vi "LSMcontroller_v62_updatedpointscan.vi"() -> ()   [LabVIEW 2015] (continued)
                                n1312 = Unbundle By Name(w3824) -> ("autoshutter"=w3823:bool, "wavdet"=w3819:bool)
                                n1313 = case shown="False" w3823 {
                                tunnel: [w3829 w3849] -> w3822
                                tunnel: [w3828 FALSE ("removal")] -> w3821
                                tunnel: [w3827 w3847] -> w3820
                                tunnel: w3819 -> [w3826 _]
                                frame False {
                                n1314 = case shown="False" w3826 {
                                tunnel: [FALSE ("addition") FALSE ("addition")] -> w3829
                                tunnel: [w3831 FALSE ("removal")] -> w3828
                                tunnel: [w3830 _] -> w3827
                                frame False {
                                n1315 = call "configuration.vi"("command"="get") -> ("config out"=w3837:T11)  [unwired: 2 in, 1 out]
                                n1316 = Unbundle By Name(w3837) -> ("2P shutter"=w3834:i32)
                                n1317 = call "2pparameters.vi"("command"="get") -> ("params out"=w3835:T10)  [unwired: 1 in]
                                n1318 = in-place {
                                in-place-border: w3834 -> [w3844]
                                in-place-border: [w3841] -> w3831
                                in-place-border: [w3840] -> w3830
                                n1319 = in-place-cluster #25(w3835) -> ("aDO"=w3843:u32[])
                                n1320 = call "remove channel from active arrayv2.vi"("line array in"=w3843, "line to remove"=w3844) -> ("line array out"=w3842:u32[], "removal"=w3841:bool, "index"=w3840:i32)
                                n1321 = in-place-cluster #25("aDO"=w3842) -> (w3832:T10)
                                }
                                n1322 = call "2pparameters.vi"("Params in"=w3832, "command"="set") -> ()  [unwired: 1 out]
                                }
                                frame True {
                                }
                                }
                                }
                                frame True {
                                n1323 = call "configuration.vi"("command"="get") -> ("config out"=w3851:T11)  [unwired: 2 in, 1 out]
                                n1324 = call "2pparameters.vi"("command"="get") -> ("params out"=w3855:T10)  [unwired: 1 in]
                                n1325 = Unbundle By Name(w3851) -> ("2P shutter"=w3850:i32)
                                n1326 = in-place {
                                in-place-border: w3850 -> [w3861]
                                in-place-border: [w3858] -> w3849
                                in-place-border: [w3857] -> w3847
                                n1327 = in-place-cluster #26(w3855) -> ("aDO"=w3860:u32[])
                                n1328 = call "add channel to active arrayv2.vi"("line array in"=w3860, "line to add"=w3861) -> ("line array out"=w3859:u32[], "addition"=w3858:bool, "index"=w3857:i32)
                                n1329 = in-place-cluster #26("aDO"=w3859) -> (w3853:T10)
                                }
                                n1330 = call "2pparameters.vi"("Params in"=w3853, "command"="set") -> ()  [unwired: 1 out]
                                }
                                }
                                }
                                frame #3 {
                                n1331 = local read "Measurement"() -> (w3865:T4)
                                n1332 = To Unsigned Long Integer(number=w3865) -> (unsigned 32bit integer=w3866:u32)
                                n1333 = case shown="5..7" w3866 {
                                tunnel: [FALSE ("addition") w3884] -> w3864
                                tunnel: [w3869 FALSE ("removal")] -> w3863
                                tunnel: [w3867 w3882] -> w3862
                                frame 0..4, Default {
                                n1334 = call "configuration.vi"("command"="get") -> ("config out"=w3875:T11)  [unwired: 2 in, 1 out]
                                n1335 = Unbundle By Name(w3875) -> ("LT timestamp"=w3872:u32)
                                n1336 = call "2pparameters.vi"("command"="get") -> ("params out"=w3873:T10)  [unwired: 1 in]
                                n1337 = in-place {
                                in-place-border: w3872 -> [w3881]
                                in-place-border: [w3878] -> w3869
                                in-place-border: [w3877] -> w3867
                                n1338 = in-place-cluster #27(w3873) -> ("aDO"=w3880:u32[])
                                n1339 = call "remove channel from active arrayv2.vi"("line array in"=w3880, "line to remove"=w3881) -> ("line array out"=w3879:u32[], "removal"=w3878:bool, "index"=w3877:i32)
                                n1340 = in-place-cluster #27("aDO"=w3879) -> (w3870:T10)
                                }
                                n1341 = call "2pparameters.vi"("Params in"=w3870, "command"="set") -> ()  [unwired: 1 out]
                                }
                                frame 5..7 {
                                n1342 = call "configuration.vi"("command"="get") -> ("config out"=w3890:T11)  [unwired: 2 in, 1 out]
                                n1343 = Unbundle By Name(w3890) -> ("LT timestamp"=w3887:u32)
                                n1344 = call "2pparameters.vi"("command"="get") -> ("params out"=w3888:T10)  [unwired: 1 in]
                                n1345 = in-place {
                                in-place-border: w3887 -> [w3896]
                                in-place-border: [w3893] -> w3884
                                in-place-border: [w3892] -> w3882
                                n1346 = in-place-cluster #28(w3888) -> ("aDO"=w3895:u32[])
                                n1347 = call "add channel to active arrayv2.vi"("line array in"=w3895, "line to add"=w3896) -> ("line array out"=w3894:u32[], "addition"=w3893:bool, "index"=w3892:i32)
                                n1348 = in-place-cluster #28("aDO"=w3894) -> (w3885:T10)
                                }
                                n1349 = call "2pparameters.vi"("Params in"=w3885, "command"="set") -> ()  [unwired: 1 out]
                                }
                                }
                                }
                                }
                                }
                                frame #1 {
                                n1350 = Or(x=w3903, y=w3904) -> (x .or. y?=w3902:bool)
                                n1351 = case shown="True" w3902 {
                                frame False {
                                }
                                frame True {
                                # "update GUI"
                                n1352 = call "Used AO lines.vi"() -> ("used AO names"=w3908:string[], "used AO lines"=w3910:tag[])  [unwired: 2 in]
                                n1353 = control-ref of="Analog Lines Plot"() -> (w3909:refnum<vi>)
                                n1354 = local write "Analog Used Lines"(w3910) -> ()
                                n1355 = local write "Analog Used Names"(w3908) -> ()
                                n1356 = call "prepAOWaveplot.vi"("WaveformGraph in"=w3909, "Analog Used Names"=w3908) -> ()  [unwired: 1 in]
                                }
                                }
                                n1357 = Compound Arithmetic op=OR(w3900, w3899, w3898, w3897) -> (w3901:bool)
                                n1358 = case shown="True" w3901 {
                                frame False {
                                }
                                frame True {
                                n1359 = control-ref of="Digital Lines Plot"() -> (w3905:refnum<vi>)
                                n1360 = call "Used DO lines.vi"() -> ("used DO names"=w3906:string[], "used DO lines"=w3907:tag[])  [unwired: 2 in]
                                n1361 = local write "Digital Used Lines"(w3907) -> ()
                                n1362 = local write "Digital Used Names"(w3906) -> ()
                                n1363 = call "prepDOWaveplot.vi"("DigitalGraph in"=w3905, "used DO names"=w3906) -> ()  [unwired: 1 in]
                                }
                                }
                                }
                                frame #2 {
                                n1364 = case shown="False" w3914 {
                                tunnel: [w3917 w3943] -> w3913
                                tunnel: [w3916 w3941] -> w3912
                                tunnel: [w3915 _] -> w3911
                                frame False {
                                n1365 = stacked-sequence {
                                seq-local: [w3919 _] -> [_ w3934]
                                tunnel: [w3919 _] -> w3917
                                tunnel: [w3922 _] -> w3916
                                tunnel: [w3918 _] -> w3915
                                frame #0 {
                                n1366 = call "configuration.vi"("command"="get") -> ("config out"=w3930:T11)  [unwired: 2 in, 1 out]
                                n1367 = call "waveformparamsv2.vi"("command"="get") -> ("Params out"=w3924:T14)  [unwired: 4 in, 2 out]
                                n1368 = Unbundle By Name(w3930) -> ("Voltage to Xgalvo"=w3931:i32)
                                n1369 = call "2pparameters.vi"("command"="get") -> ("params out"=w3927:T10)  [unwired: 1 in]
                                n1370 = Unbundle By Name(w3924) -> ("AO parameters"=w3923:T15)
                                n1371 = Unbundle By Name(w3927) -> ("aAO"=w3928:u32[])
                                n1372 = call "waveformsAObuffer.vi"("command"="get") -> ("AO wf out"=w3920:waveform(dbl)[])  [unwired: 1 in]
                                n1373 = Search 1D Array(1D array=w3928, element=w3931) -> (index of element=w3919:i32)  [unwired: 1 in]
                                n1374 = Index Array(array=w3920, index=w3919) -> (element=w3918:waveform(dbl))
                                n1375 = Index Array(array=w3923, index=w3919) -> (element=w3922:T16)
                                }
                                frame #1 {
                                w3935 = 0.0 ("Step size (V)")
                                n1376 = local read "Meastab"() -> (w3933:enum32{"X-Y Image", "Linescan", "Timetrace"})
                                n1377 = case shown="\"X-Y Image\", Default" w3933 {
                                tunnel: [w3937 w3938] -> w3932
                                frame "X-Y Image", Default {
                                n1378 = local read "Sampling rate"() -> (w3937:dbl)
                                }
                                frame "Timetrace" {
                                n1379 = local read "srateAODOtt"() -> (w3938:dbl)
                                }
                                }
                                n1380 = call "replace AO XYwfparam.vi"("Baseline (V)"=w3935, "Start amplitude (V)"=w3935, "Cycles"=w3935, "Repeats"=w3935, "index of AO wave"=w3934, "Step size (V)"=w3935, "DC (%)"=w3935, "Sampling frequency (Hz)"=w3932, "Period (ms)"=w3935, "Cycle length (s)"=w3935, "Pulses"=w3935, "padding value"=w3935, "Matlab wave name"=path "xwave") -> ()  [unwired: 3 in]
                                }
                                }
                                }
                                frame True {
                                w3942 = 0.0 ("Repeats")
                                n1381 = local read "Meastab"() -> (w3940:enum32{"X-Y Image", "Linescan", "Timetrace"})
                                n1382 = case shown="\"X-Y Image\", Default" w3940 {
                                tunnel: [w3959 w3960] -> w3939
                                frame "X-Y Image", Default {
                                n1383 = local read "Sampling rate"() -> (w3959:dbl)
                                }
                                frame "Timetrace" {
                                n1384 = local read "srateAODOtt"() -> (w3960:dbl)
                                }
                                }
                                n1385 = call "2pparameters.vi"("command"="get") -> ("params out"=w3945:T10)  [unwired: 1 in]
                                n1386 = call "configuration.vi"("command"="get") -> ("config out"=w3948:T11)  [unwired: 2 in, 1 out]
                                n1387 = call "waveformparamsv2.vi"("command"="get") -> ("Params out"=w3956:T14)  [unwired: 4 in, 2 out]
                                n1388 = Unbundle By Name(w3948) -> ("Voltage to Xgalvo"=w3949:i32)
                                n1389 = Unbundle By Name(w3956) -> ("AO parameters"=w3953:T15)
                                n1390 = Unbundle By Name(w3945) -> ("aAO"=w3946:u32[])
                                n1391 = Search 1D Array(1D array=w3946, element=w3949) -> (index of element=w3943:i32)  [unwired: 1 in]
                                n1392 = Index Array(array=w3953, index=0) -> (element=w3954:T16)
                                n1393 = Bundle By Name(cluster=w3954, "AOtab"=-1.0 ("Repeats"), "Repeats"=w3942, "Cycles"=w3942, "Start amplitude (V)"=w3942, "Baseline (V)"=w3942, "Step size (V)"=w3942, "DC (%)"=w3942, "Sampling frequency (Hz)"=w3939, "Period (ms)"=w3942, "Offset (V)"=w3942, "Amplitude (V)"=w3942, "Frequency"=w3942, "Tri Repeats"=w3942, "phase shift (ms)"=w3942, "Pulses"=w3942, "Matlab wave file"=path "xwave", "padding value"=w3942) -> (w3941:T16)
                                n1394 = Build Array(w3941) -> (w3951:T15)
                                n1395 = call "waveformparamsv2.vi"("command"="add AO", "add AO"=w3951) -> ()  [unwired: 3 in, 3 out]
                                }
                                }
                                }
                                frame #3 {
                                n1396 = case shown="False" w3964 {
                                tunnel: [w3967 w3993] -> w3963
                                tunnel: [w3966 w3991] -> w3962
                                tunnel: [w3965 _] -> w3961
                                frame False {
                                n1397 = stacked-sequence {
                                seq-local: [w3969 _] -> [_ w3984]
                                tunnel: [w3969 _] -> w3967
                                tunnel: [w3972 _] -> w3966
                                tunnel: [w3968 _] -> w3965
                                frame #0 {
                                n1398 = call "configuration.vi"("command"="get") -> ("config out"=w3980:T11)  [unwired: 2 in, 1 out]
                                n1399 = call "waveformparamsv2.vi"("command"="get") -> ("Params out"=w3974:T14)  [unwired: 4 in, 2 out]
                                n1400 = Unbundle By Name(w3980) -> ("Voltage to Ygalvo"=w3981:i32)
                                n1401 = call "2pparameters.vi"("command"="get") -> ("params out"=w3977:T10)  [unwired: 1 in]
                                n1402 = Unbundle By Name(w3974) -> ("AO parameters"=w3973:T15)
                                n1403 = Unbundle By Name(w3977) -> ("aAO"=w3978:u32[])
                                n1404 = call "waveformsAObuffer.vi"("command"="get") -> ("AO wf out"=w3970:waveform(dbl)[])  [unwired: 1 in]
                                n1405 = Search 1D Array(1D array=w3978, element=w3981) -> (index of element=w3969:i32)  [unwired: 1 in]
                                n1406 = Index Array(array=w3970, index=w3969) -> (element=w3968:waveform(dbl))
                                n1407 = Index Array(array=w3973, index=w3969) -> (element=w3972:T16)
                                }
                                frame #1 {
                                w3985 = 0.0 ("Step size (V)")
                                n1408 = local read "Meastab"() -> (w3983:enum32{"X-Y Image", "Linescan", "Timetrace"})
                                n1409 = case shown="\"X-Y Image\", Default" w3983 {
                                tunnel: [w3987 w3988] -> w3982
                                frame "X-Y Image", Default {
                                n1410 = local read "Sampling rate"() -> (w3987:dbl)
                                }
                                frame "Timetrace" {
                                n1411 = local read "srateAODOtt"() -> (w3988:dbl)
                                }
                                }
                                n1412 = call "replace AO XYwfparam.vi"("Baseline (V)"=w3985, "Start amplitude (V)"=w3985, "Cycles"=w3985, "Repeats"=w3985, "index of AO wave"=w3984, "Step size (V)"=w3985, "DC (%)"=w3985, "Sampling frequency (Hz)"=w3982, "Period (ms)"=w3985, "Cycle length (s)"=w3985, "Pulses"=w3985, "padding value"=w3985, "Matlab wave name"=path "ywave") -> ()  [unwired: 3 in]
                                }
                                }
                                }
                                frame True {
                                w3992 = 0.0 ("Repeats")
                                n1413 = local read "Meastab"() -> (w3990:enum32{"X-Y Image", "Linescan", "Timetrace"})
                                n1414 = case shown="\"X-Y Image\", Default" w3990 {
                                tunnel: [w4009 w4010] -> w3989
                                frame "X-Y Image", Default {
                                n1415 = local read "Sampling rate"() -> (w4009:dbl)
                                }
                                frame "Timetrace" {
                                n1416 = local read "srateAODOtt"() -> (w4010:dbl)
                                }
                                }
                                n1417 = call "2pparameters.vi"("command"="get") -> ("params out"=w3995:T10)  [unwired: 1 in]
                                n1418 = call "configuration.vi"("command"="get") -> ("config out"=w3998:T11)  [unwired: 2 in, 1 out]
                                n1419 = call "waveformparamsv2.vi"("command"="get") -> ("Params out"=w4007:T14)  [unwired: 4 in, 2 out]
                                n1420 = Unbundle By Name(w3998) -> ("Voltage to Ygalvo"=w3999:i32)
                                n1421 = Unbundle By Name(w4007) -> ("AO parameters"=w4004:T15)
                                n1422 = Unbundle By Name(w3995) -> ("aAO"=w3996:u32[])
                                n1423 = Search 1D Array(1D array=w3996, element=w3999) -> (index of element=w3993:i32)  [unwired: 1 in]
                                n1424 = Index Array(array=w4004, index=0) -> (element=w4005:T16)
                                n1425 = Bundle By Name(cluster=w4005, "AOtab"=-1.0 ("Repeats"), "Repeats"=w3992, "Cycles"=w3992, "Start amplitude (V)"=w3992, "Baseline (V)"=w3992, "Step size (V)"=w3992, "DC (%)"=w3992, "Sampling frequency (Hz)"=w3989, "Period (ms)"=w3992, "Offset (V)"=w3992, "Amplitude (V)"=w3992, "Frequency"=w3992, "Tri Repeats"=w3992, "phase shift (ms)"=w3992, "Pulses"=w3992, "Matlab wave file"=path "ywave", "padding value"=w3992) -> (w3991:T16)
                                n1426 = Build Array(w3991) -> (w4002:T15)
                                n1427 = call "waveformparamsv2.vi"("command"="add AO", "add AO"=w4002) -> ()  [unwired: 3 in, 3 out]
                                }
                                }
                                }
                                frame #4 {
                                n1428 = call "2pparameters.vi"("command"="get") -> ("params out"=w4016:T10)  [unwired: 1 in]
                                n1429 = Unbundle By Name(w4016) -> ("wavdet"=w4015:bool, "Pel"=w4012:sgl, "refwfsize"=w4011:dbl, "srateAODO"=w4014:sgl)
                                n1430 = case shown="True" w4015 {
                                tunnel: [w4020 w4030] -> w4018
                                tunnel: w4014 -> [w4021 w4032]
                                tunnel: w4012 -> [_ w4028]
                                tunnel: w4011 -> [_ w4027]
                                frame False {
                                n1431 = call "X-array-databuffer.vi"("command"=enum16{"get", "set", "clear", "append"}."get") -> ("array out"=w4024:dbl[])  [unwired: 3 in, 1 out]
                                n1432 = Reciprocal(x=w4021) -> (1/x=w4022:sgl)
                                n1433 = Bundle By Name("Y"=w4024, "dt"=w4022) -> (w4020:waveform(dbl))  [unwired: 1 in]
                                }
                                frame True {
                                n1434 = To Double Precision Float(number=w4028) -> (double precision float=w4029:dbl)
                                n1435 = Divide(x=w4027, y=w4029) -> (x/y=w4026:dbl)
                                n1436 = Round Toward +Infinity(x=w4026) -> (ceil(x): smallest int >= x=w4025:dbl)
                                n1437 = call "X-array-databuffer.vi"("command"=enum16{"get", "set", "clear", "append"}."get") -> ("array out"=w4034:dbl[])  [unwired: 3 in, 1 out]
                                n1438 = Reciprocal(x=w4032) -> (1/x=w4033:sgl)
                                n1439 = for {
                                N: w4025 -> [_]
                                tunnel: w4034 -> [w4036]
                                tunnel: [w4036] -> w4031 mode=concatenating
                                }
                                n1440 = Bundle By Name("Y"=w4031, "dt"=w4033) -> (w4030:waveform(dbl))  [unwired: 1 in]
                                }
                                }
                                n1441 = case shown="True" w4019 {
                                tunnel: w4018 -> [w4038 w4044]
                                tunnel: w4013 -> [w4039 _]
                                frame False {
                                n1442 = call "waveformsAObuffer.vi"("command"="get") -> ("AO wf out"=w4042:waveform(dbl)[])  [unwired: 1 in]
                                n1443 = property on="refwf" class="Ring (strict)" props=["RingText", "Text"]() -> ()  [unwired: 2 in, 3 out]
                                n1444 = Replace Array Subset(array=w4042, new element=w4038, index=w4039) -> (w4037:waveform(dbl)[])
                                n1445 = call "waveformsAObuffer.vi"("AO wf in"=w4037, "command"="set") -> ()  [unwired: 1 out]
                                }
                                frame True {
                                n1446 = call "waveformsAObuffer.vi"("command"="get") -> ("AO wf out"=w4046:waveform(dbl)[])  [unwired: 1 in]
                                n1447 = Build Array (concatenate)(w4046, w4044) -> (w4043:waveform(dbl)[])
                                n1448 = call "waveformsAObuffer.vi"("AO wf in"=w4043, "command"="set") -> ()  [unwired: 1 out]
                                }
                                }
                                }
                                frame #5 {
                                n1449 = call "2pparameters.vi"("command"="get") -> ("params out"=w4058:T10)  [unwired: 1 in]
                                n1450 = Unbundle By Name(w4058) -> ("wavdet"=w4057:bool, "Pel"=w4055:sgl, "refwfsize"=w4056:dbl, "srateAODO"=w4051:sgl)
                                n1451 = To Double Precision Float(number=w4055) -> (double precision float=w4054:dbl)
                                n1452 = Divide(x=w4056, y=w4054) -> (x/y=w4053:dbl)
                                n1453 = Round Toward +Infinity(x=w4053) -> (ceil(x): smallest int >= x=w4052:dbl)
                                n1454 = case shown="True" w4057 {
                                tunnel: [w4062 w4068] -> w4048
                                tunnel: w4052 -> [_ w4065]
                                tunnel: w4051 -> [w4063 w4070]
                                frame False {
                                n1455 = call "Y-array-databuffer.vi"("command"=enum16{"get", "set", "clear", "append"}."get") -> ("array out"=w4060:dbl[])  [unwired: 3 in, 1 out]
                                n1456 = Reciprocal(x=w4063) -> (1/x=w4064:sgl)
                                n1457 = Bundle By Name("Y"=w4060, "dt"=w4064) -> (w4062:waveform(dbl))  [unwired: 1 in]
                                }
                                frame True {
                                n1458 = call "Y-array-databuffer.vi"("command"=enum16{"get", "set", "clear", "append"}."get") -> ("array out"=w4066:dbl[])  [unwired: 3 in, 1 out]
                                n1459 = Reciprocal(x=w4070) -> (1/x=w4071:sgl)
                                n1460 = for {
                                N: w4065 -> [_]
                                tunnel: w4066 -> [w4072]
                                tunnel: [w4072] -> w4069 mode=concatenating
                                }
                                n1461 = Bundle By Name("Y"=w4069, "dt"=w4071) -> (w4068:waveform(dbl))  [unwired: 1 in]
                                }
                                }
                                n1462 = case shown="False" w4050 {
                                tunnel: w4048 -> [w4075 w4080]
                                tunnel: w4049 -> [w4076 _]
                                frame False {
                                n1463 = call "waveformsAObuffer.vi"("command"="get") -> ("AO wf out"=w4078:waveform(dbl)[])  [unwired: 1 in]
                                n1464 = Replace Array Subset(array=w4078, new element=w4075, index=w4076) -> (w4073:waveform(dbl)[])
                                n1465 = call "waveformsAObuffer.vi"("AO wf in"=w4073, "command"="set") -> ()  [unwired: 1 out]
                                }
                                frame True {
                                n1466 = call "waveformsAObuffer.vi"("command"="get") -> ("AO wf out"=w4082:waveform(dbl)[])  [unwired: 1 in]
                                n1467 = Build Array (concatenate)(w4082, w4080) -> (w4079:waveform(dbl)[])
                                n1468 = call "waveformsAObuffer.vi"("AO wf in"=w4079, "command"="set") -> ()  [unwired: 1 out]
                                }
                                }
                                }
                                frame #6 {
                                n1469 = Build Array(w4087, w4086) -> (w4090:bool[])
                                n1470 = Boolean Array To Number(Boolean array=w4090) -> (number=w4089:u32)
                                n1471 = case shown="2" w4089 {
                                tunnel: w4088 -> [_ _ _ _]
                                tunnel: w4085 -> [_ w4113 _ w4126]
                                tunnel: [_ w4112 _ w4123] -> w4084
                                frame 1 {
                                w4100 = 0.0 ("DOtab")
                                n1472 = call "2pparameters.vi"("command"="get") -> ("params out"=w4097:T10)  [unwired: 1 in]
                                n1473 = call "waveformparamsv2.vi"("command"="get") -> ("Params out"=w4108:T14)  [unwired: 4 in, 2 out]
                                n1474 = Unbundle By Name(w4108) -> ("DO parameters"=w4106:T17)
                                n1475 = Unbundle By Name(w4097) -> ("srate"=w4093:sgl, "Pel"=w4096:sgl)
                                n1476 = To Double Precision Float(number=w4093) -> (double precision float=w4091:dbl)
                                n1477 = To Double Precision Float(number=w4093) -> (double precision float=w4092:dbl)
                                n1478 = To Double Precision Float(number=w4096) -> (double precision float=w4095:dbl)
                                n1479 = Divide(x=w4092, y=w4095) -> (x/y=w4094:dbl)
                                n1480 = Index Array(array=w4106, index=0) -> (element=w4105:T18)
                                n1481 = Bundle By Name(cluster=w4105, "Digital DC (%)"=100.0, "Digital phase"=w4100, "Digital Freq (Hz)"=w4094, "Sampling frequency (Hz)"=w4091, "Digital time offset (s)"=w4100, "padding value"=0.0, "matlab wave file"=path "2Pshutter", "DOtab"=0.0) -> (w4103:T18)
                                n1482 = Build Array(w4103) -> (w4102:T17)
                                n1483 = call "waveformparamsv2.vi"("command"="add DO", "add DO"=w4102) -> ()  [unwired: 3 in, 3 out]
                                }
                                frame 2 {
                                n1484 = call "waveformparamsv2.vi"("command"="get") -> ("Params out"=w4115:T14)  [unwired: 4 in, 2 out]
                                n1485 = in-place {
                                in-place-border: w4113 -> [w4119]
                                in-place-border: [w4118] -> w4112
                                n1486 = in-place-cluster #29(w4115) -> ("DO parameters"=w4121:T17)
                                n1487 = Delete From Array(array=w4121, length=1, index=w4119) -> (deleted portion=w4118:T17, array with subset deleted=w4120:T17)
                                n1488 = in-place-cluster #29("DO parameters"=w4120) -> (w4114:T14)
                                }
                                n1489 = call "waveformparamsv2.vi"("command"="set", "Params in"=w4114) -> ()  [unwired: 3 in, 3 out]
                                }
                                frame 3, Default {
                                }
                                frame 0 {
                                n1490 = call "2pparameters.vi"("command"="get") -> ("params out"=w4128:T10)  [unwired: 1 in]
                                n1491 = Unbundle By Name(w4128) -> ("wavdet"=w4125:bool, "autoshutter"=w4127:bool)
                                n1492 = case shown="True" w4127 {
                                tunnel: w4126 -> [_ w4132]
                                tunnel: w4125 -> [_ w4131]
                                tunnel: [_ w4130] -> w4124
                                frame False {
                                }
                                frame True {
                                n1493 = case shown="False" w4131 {
                                tunnel: w4132 -> [w4134 _]
                                tunnel: [w4133 _] -> w4130
                                frame False {
                                n1494 = stacked-sequence {
                                tunnel: w4134 -> [w4136 w4150]
                                tunnel: [w4135 _] -> w4133
                                frame #0 {
                                n1495 = call "waveformparamsv2.vi"("command"="get") -> ("Params out"=w4138:T14)  [unwired: 4 in, 2 out]
                                n1496 = Unbundle By Name(w4138) -> ("DO parameters"=w4137:T17)
                                n1497 = Index Array(array=w4137, index=w4136) -> (element=w4135:T18)
                                }
                                frame #1 {
                                w4149 = 0.0 ("padding value")
                                n1498 = call "2pparameters.vi"("command"="get") -> ("params out"=w4147:T10)  [unwired: 1 in]
                                n1499 = Unbundle By Name(w4147) -> ("srate"=w4144:sgl, "Pel"=w4146:sgl)
                                n1500 = To Double Precision Float(number=w4144) -> (double precision float=w4142:dbl)
                                n1501 = To Double Precision Float(number=w4144) -> (double precision float=w4143:dbl)
                                n1502 = To Double Precision Float(number=w4146) -> (double precision float=w4145:dbl)
                                n1503 = Divide(x=w4143, y=w4145) -> (x/y=w4141:dbl)
                                n1504 = call "replace DO wf param.vi"("Digital Freq (Hz)"=w4141, "Digital DC (%)"=100.0, "Digital phase"=w4149, "Sampling frequency (Hz)"=w4142, "Digital time offset (s)"=w4149, "index of DO wave"=w4150, "padding value"=w4149, "matlab wave file"=path "2Pshutter" ("matlab wave number")) -> ()  [unwired: 3 in]
                                }
                                }
                                }
                                frame True {
                                }
                                }
                                }
                                }
                                n1505 = Build Array(w4124) -> (w4123:T17)
                                }
                                }
                                }
                                frame #7 {
                                n1506 = Build Array(w4155, w4154) -> (w4157:bool[])
                                n1507 = Boolean Array To Number(Boolean array=w4157) -> (number=w4156:u32)
                                n1508 = case shown="0" w4156 {
                                tunnel: w4153 -> [_ w4199 _ w4206]
                                tunnel: [_ w4198 _ w4204] -> w4152
                                frame 1 {
                                n1509 = call "2pparameters.vi"("command"="get") -> ("params out"=w4164:T10)  [unwired: 1 in]
                                n1510 = Unbundle By Name(w4164) -> ("wavdet"=w4165:bool, "Pel"=w4167:sgl, "refwfsize"=w4168:dbl, "srateAODO"=w4166:sgl)
                                n1511 = call "waveformsDObuffer.vi"("command"="get") -> ("DO wf out"=w4160:digitalwaveform[])  [unwired: 1 in]
                                n1512 = case shown="False" w4165 {
                                tunnel: [w4173 w4183] -> w4162
                                tunnel: w4166 -> [w4178 w4194]
                                tunnel: w4167 -> [w4172 w4187]
                                tunnel: w4168 -> [_ w4191]
                                frame False {
                                w4176 = u16 0 items=["unsigned binary", "offset binary", "2's complement"] ("data format (offset binary)")
                                n1513 = Initialize Array(sgl 1.0, w4172) -> (w4169:sgl[])
                                n1514 = Reciprocal(x=w4178) -> (1/x=w4179:sgl)
                                n1515 = Bundle By Name("Y"=w4169, "dt"=w4179) -> (w4174:waveform(sgl))  [unwired: 1 in]
                                n1516 = call-poly <vilib>:"Analog to Digital.vi"("data format (offset binary)"=w4176, "compress digital (T)"=TRUE, "full-scale range (pk-pk)"=1.0, "resolution (16 bit)"=1, "analog waveform"=w4174) -> ("digital waveform"=w4173:digitalwaveform)  [unwired: 3 in, 3 out]
                                }
                                frame True {
                                w4186 = u16 0 items=["unsigned binary", "offset binary", "2's complement"] ("data format (offset binary)")
                                n1517 = To Double Precision Float(number=w4187) -> (double precision float=w4192:dbl)
                                n1518 = Initialize Array(sgl 1.0, w4187) -> (w4180:sgl[])
                                n1519 = Divide(x=w4191, y=w4192) -> (x/y=w4189:dbl)
                                n1520 = Round Toward +Infinity(x=w4189) -> (ceil(x): smallest int >= x=w4190:dbl)
                                n1521 = for {
                                N: w4190 -> [_]
                                tunnel: w4180 -> [w4196]
                                tunnel: [w4196] -> w4193 mode=concatenating
                                }
                                n1522 = Reciprocal(x=w4194) -> (1/x=w4195:sgl)
                                n1523 = Bundle By Name("Y"=w4193, "dt"=w4195) -> (w4184:waveform(sgl))  [unwired: 1 in]
                                n1524 = call-poly <vilib>:"Analog to Digital.vi"("data format (offset binary)"=w4186, "compress digital (T)"=TRUE, "full-scale range (pk-pk)"=1.0, "resolution (16 bit)"=1, "analog waveform"=w4184) -> ("digital waveform"=w4183:digitalwaveform)  [unwired: 3 in, 3 out]
                                }
                                }
                                n1525 = Build Array (concatenate)(w4160, w4162) -> (w4158:digitalwaveform[])
                                n1526 = call "waveformsDObuffer.vi"("DO wf in"=w4158, "command"="set") -> ()  [unwired: 1 out]
                                }
                                frame 2 {
                                n1527 = call "waveformsDObuffer.vi"("command"="get") -> ("DO wf out"=w4201:digitalwaveform[])  [unwired: 1 in]
                                n1528 = Delete From Array(array=w4201, length=1, index=w4199) -> (deleted portion=w4198:digitalwaveform[], array with subset deleted=w4197:digitalwaveform[])
                                n1529 = call "waveformsDObuffer.vi"("DO wf in"=w4197, "command"="set") -> ()  [unwired: 1 out]
                                }
                                frame 3, Default {
                                }
                                frame 0 {
                                n1530 = call "2pparameters.vi"("command"="get") -> ("params out"=w4208:T10)  [unwired: 1 in]
                                n1531 = Unbundle By Name(w4208) -> ("autoshutter"=w4207:bool, "wavdet"=w4205:bool)
                                n1532 = case shown="True" w4207 {
                                tunnel: w4206 -> [_ w4212]
                                tunnel: w4205 -> [_ w4211]
                                tunnel: [_ w4210] -> w4204
                                frame False {
                                }
                                frame True {
                                n1533 = case shown="False" w4211 {
                                tunnel: w4212 -> [w4216 _]
                                tunnel: [w4214 _] -> w4210
                                frame False {
                                w4223 = u16 0 items=["unsigned binary", "offset binary", "2's complement"] ("data format (offset binary)")
                                n1534 = call "2pparameters.vi"("command"="get") -> ("params out"=w4230:T10)  [unwired: 1 in]
                                n1535 = call "waveformsDObuffer.vi"("command"="get") -> ("DO wf out"=w4217:digitalwaveform[])  [unwired: 1 in]
                                n1536 = Unbundle By Name(w4230) -> ("Pel"=w4232:sgl, "srate"=w4231:sgl)
                                n1537 = Index Array(array=w4217, index=w4216) -> (element=w4215:digitalwaveform)
                                n1538 = Build Array(w4215) -> (w4214:digitalwaveform[])
                                n1539 = Initialize Array(sgl 1.0, w4232) -> (w4218:sgl[])
                                n1540 = Reciprocal(x=w4231) -> (1/x=w4225:sgl)
                                n1541 = Bundle By Name("Y"=w4218, "dt"=w4225) -> (w4221:waveform(sgl))  [unwired: 1 in]
                                n1542 = call-poly <vilib>:"Analog to Digital.vi"("data format (offset binary)"=w4223, "compress digital (T)"=TRUE, "full-scale range (pk-pk)"=1.0, "resolution (16 bit)"=1, "analog waveform"=w4221) -> ("digital waveform"=w4228:digitalwaveform)  [unwired: 3 in, 3 out]
                                n1543 = Replace Array Subset(array=w4217, new element=w4228, index=w4216) -> (w4213:digitalwaveform[])
                                n1544 = call "waveformsDObuffer.vi"("DO wf in"=w4213, "command"="set") -> ()  [unwired: 1 out]
                                }
                                frame True {
                                }
                                }
                                }
                                }
                                }
                                }
                                }
                                frame #8 {
                                n1545 = Build Array(w4236, w4235) -> (w4238:bool[])
                                n1546 = Boolean Array To Number(Boolean array=w4238) -> (number=w4237:u32)
                                n1547 = case shown="0" w4237 {
                                tunnel: w4234 -> [_ w4264 _ w4276]
                                tunnel: [_ w4263 _ w4274] -> w4233
                                frame 1 {
                                w4251 = 0.0 ("DOtab")
                                n1548 = call "2pparameters.vi"("command"="get") -> ("params out"=w4249:T10)  [unwired: 1 in]
                                n1549 = call "waveformparamsv2.vi"("command"="get") -> ("Params out"=w4259:T14)  [unwired: 4 in, 2 out]
                                n1550 = Unbundle By Name(w4259) -> ("DO parameters"=w4257:T17)
                                n1551 = Unbundle By Name(w4249) -> ("srate"=w4246:sgl, "Pel"=w4248:sgl)
                                n1552 = To Double Precision Float(number=w4246) -> (double precision float=w4244:dbl)
                                n1553 = To Double Precision Float(number=w4246) -> (double precision float=w4245:dbl)
                                n1554 = To Double Precision Float(number=w4248) -> (double precision float=w4240:dbl)
                                n1555 = Divide(x=w4245, y=w4240) -> (x/y=w4247:dbl)
                                n1556 = Index Array(array=w4257, index=0) -> (element=w4256:T18)
                                n1557 = Divide(x=1.0 ("Digital DC (%)"), y=w4240) -> (x/y=w4242:dbl)
                                n1558 = Multiply(x=100.0, y=w4242) -> (x*y=w4239:dbl)
                                n1559 = Bundle By Name(cluster=w4256, "Digital DC (%)"=w4239, "Digital phase"=w4251, "Digital Freq (Hz)"=w4247, "Sampling frequency (Hz)"=w4244, "Digital time offset (s)"=w4251, "padding value"=0.0, "matlab wave file"=path "LT", "DOtab"=0.0) -> (w4254:T18)
                                n1560 = Build Array(w4254) -> (w4253:T17)
                                n1561 = call "waveformparamsv2.vi"("command"="add DO", "add DO"=w4253) -> ()  [unwired: 3 in, 3 out]
                                }
                                frame 2 {
                                n1562 = call "waveformparamsv2.vi"("command"="get") -> ("Params out"=w4266:T14)  [unwired: 4 in, 2 out]
                                n1563 = in-place {
                                in-place-border: w4264 -> [w4270]
                                in-place-border: [w4269] -> w4263
                                n1564 = in-place-cluster #30(w4266) -> ("DO parameters"=w4272:T17)
                                n1565 = Delete From Array(array=w4272, length=1, index=w4270) -> (deleted portion=w4269:T17, array with subset deleted=w4271:T17)
                                n1566 = in-place-cluster #30("DO parameters"=w4271) -> (w4265:T14)
                                }
                                n1567 = call "waveformparamsv2.vi"("command"="set", "Params in"=w4265) -> ()  [unwired: 3 in, 3 out]
                                }
                                frame 3, Default {
                                }
                                frame 0 {
                                n1568 = local read "Measurement"() -> (w4278:T4)
                                n1569 = To Unsigned Long Integer(number=w4278) -> (unsigned 32bit integer=w4277:u32)
                                n1570 = case shown="5..7" w4277 {
                                tunnel: w4276 -> [_ w4280]
                                tunnel: [_ w4279] -> w4275
                                frame 0..4, Default {
                                }
                                frame 5..7 {
                                n1571 = stacked-sequence {
                                tunnel: w4280 -> [w4282 w4291]
                                tunnel: [w4281 _] -> w4279
                                frame #0 {
                                n1572 = call "waveformparamsv2.vi"("command"="get") -> ("Params out"=w4284:T14)  [unwired: 4 in, 2 out]
                                n1573 = Unbundle By Name(w4284) -> ("DO parameters"=w4285:T17)
                                n1574 = Index Array(array=w4285, index=w4282) -> (element=w4281:T18)
                                }
                                frame #1 {
                                w4299 = 0.0 ("padding value")
                                n1575 = call "2pparameters.vi"("command"="get") -> ("params out"=w4297:T10)  [unwired: 1 in]
                                n1576 = Unbundle By Name(w4297) -> ("srate"=w4295:sgl, "Pel"=w4296:sgl)
                                n1577 = To Double Precision Float(number=w4295) -> (double precision float=w4293:dbl)
                                n1578 = To Double Precision Float(number=w4295) -> (double precision float=w4294:dbl)
                                n1579 = To Double Precision Float(number=w4296) -> (double precision float=w4289:dbl)
                                n1580 = Divide(x=1.0 ("Digital DC (%)"), y=w4289) -> (x/y=w4288:dbl)
                                n1581 = Multiply(x=100.0, y=w4288) -> (x*y=w4287:dbl)
                                n1582 = Divide(x=w4294, y=w4289) -> (x/y=w4292:dbl)
                                n1583 = call "replace DO wf param.vi"("Digital Freq (Hz)"=w4292, "Digital DC (%)"=w4287, "Digital phase"=w4299, "Sampling frequency (Hz)"=w4293, "Digital time offset (s)"=w4299, "index of DO wave"=w4291, "padding value"=w4299, "matlab wave file"=path "LT" ("matlab wave number")) -> ()  [unwired: 3 in]
                                }
                                }
                                }
                                }
                                n1584 = Build Array(w4275) -> (w4274:T17)
                                }
                                }
                                }
                                frame #9 {
                                n1585 = Build Array(w4304, w4303) -> (w4306:bool[])
                                n1586 = Boolean Array To Number(Boolean array=w4306) -> (number=w4305:u32)
                                n1587 = case shown="0" w4305 {
                                tunnel: w4302 -> [_ w4358 _ w4362]
                                tunnel: [_ w4353 _ w4359] -> w4301
                                frame 1 {
                                n1588 = call "2pparameters.vi"("command"="get") -> ("params out"=w4313:T10)  [unwired: 1 in]
                                n1589 = Unbundle By Name(w4313) -> ("wavdet"=w4314:bool, "Pel"=w4316:sgl, "refwfsize"=w4317:dbl, "Pel"=w4315:sgl)
                                n1590 = call "waveformsDObuffer.vi"("command"="get") -> ("DO wf out"=w4309:digitalwaveform[])  [unwired: 1 in]
                                n1591 = case shown="True" w4314 {
                                tunnel: [w4321 w4334] -> w4311
                                tunnel: w4315 -> [w4330 w4349]
                                tunnel: w4316 -> [w4320 w4340]
                                tunnel: w4317 -> [_ w4346]
                                frame False {
                                w4324 = u16 0 items=["unsigned binary", "offset binary", "2's complement"] ("data format (offset binary)")
                                n1592 = Initialize Array(sgl 0.0, w4320) -> (w4327:sgl[])
                                n1593 = Replace Array Subset(array=w4327, new element=sgl 1.0, index=0) -> (w4325:sgl[])
                                n1594 = Reciprocal(x=w4330) -> (1/x=w4331:sgl)
                                n1595 = Bundle By Name("Y"=w4325, "dt"=w4331) -> (w4322:waveform(sgl))  [unwired: 1 in]
                                n1596 = call-poly <vilib>:"Analog to Digital.vi"("data format (offset binary)"=w4324, "compress digital (T)"=TRUE, "full-scale range (pk-pk)"=1.0, "resolution (16 bit)"=1, "analog waveform"=w4322) -> ("digital waveform"=w4321:digitalwaveform)  [unwired: 3 in, 3 out]
                                }
                                frame True {
                                w4337 = u16 0 items=["unsigned binary", "offset binary", "2's complement"] ("data format (offset binary)")
                                n1597 = To Double Precision Float(number=w4340) -> (double precision float=w4347:dbl)
                                n1598 = Initialize Array(sgl 0.0, w4340) -> (w4342:sgl[])
                                n1599 = Divide(x=w4346, y=w4347) -> (x/y=w4344:dbl)
                                n1600 = Round Toward +Infinity(x=w4344) -> (ceil(x): smallest int >= x=w4345:dbl)
                                n1601 = Replace Array Subset(array=w4342, new element=sgl 1.0, index=0) -> (w4339:sgl[])
                                n1602 = for {
                                N: w4345 -> [_]
                                tunnel: w4339 -> [w4351]
                                tunnel: [w4351] -> w4348 mode=concatenating
                                }
                                n1603 = Reciprocal(x=w4349) -> (1/x=w4350:sgl)
                                n1604 = Bundle By Name("Y"=w4348, "dt"=w4350) -> (w4335:waveform(sgl))  [unwired: 1 in]
                                n1605 = call-poly <vilib>:"Analog to Digital.vi"("data format (offset binary)"=w4337, "compress digital (T)"=TRUE, "full-scale range (pk-pk)"=1.0, "resolution (16 bit)"=1, "analog waveform"=w4335) -> ("digital waveform"=w4334:digitalwaveform)  [unwired: 3 in, 3 out]
                                }
                                }
                                n1606 = Build Array (concatenate)(w4309, w4311) -> (w4307:digitalwaveform[])
                                n1607 = call "waveformsDObuffer.vi"("DO wf in"=w4307, "command"="set") -> ()  [unwired: 1 out]
                                }
                                frame 2 {
                                n1608 = call "waveformsDObuffer.vi"("command"="get") -> ("DO wf out"=w4355:digitalwaveform[])  [unwired: 1 in]
                                n1609 = Delete From Array(array=w4355, length=1, index=w4358) -> (deleted portion=w4353:digitalwaveform[], array with subset deleted=w4352:digitalwaveform[])
                                n1610 = call "waveformsDObuffer.vi"("DO wf in"=w4352, "command"="set") -> ()  [unwired: 1 out]
                                }
                                frame 3, Default {
                                }
                                frame 0 {
                                n1611 = local read "Measurement"() -> (w4361:T4)
                                n1612 = To Unsigned Long Integer(number=w4361) -> (unsigned 32bit integer=w4360:u32)
                                n1613 = case shown="5..7" w4360 {
                                tunnel: w4362 -> [_ w4365]
                                tunnel: [_ w4364] -> w4359
                                frame 0..4, Default {
                                }
                                frame 5..7 {
                                n1614 = call "2pparameters.vi"("command"="get") -> ("params out"=w4372:T10)  [unwired: 1 in]
                                n1615 = Unbundle By Name(w4372) -> ("wavdet"=w4373:bool, "Pel"=w4375:sgl, "refwfsize"=w4376:dbl, "srateAODO"=w4374:sgl)
                                n1616 = call "waveformsDObuffer.vi"("command"="get") -> ("DO wf out"=w4366:digitalwaveform[])  [unwired: 1 in]
                                n1617 = Index Array(array=w4366, index=w4365) -> (element=w4367:digitalwaveform)
                                n1618 = case shown="True" w4373 {
                                tunnel: [w4380 w4393] -> w4370
                                tunnel: w4374 -> [w4389 w4408]
                                tunnel: w4375 -> [w4379 w4399]
                                tunnel: w4376 -> [_ w4405]
                                frame False {
                                w4383 = u16 0 items=["unsigned binary", "offset binary", "2's complement"] ("data format (offset binary)")
                                n1619 = Initialize Array(sgl 0.0, w4379) -> (w4386:sgl[])
                                n1620 = Replace Array Subset(array=w4386, new element=sgl 1.0, index=0) -> (w4384:sgl[])
                                n1621 = Reciprocal(x=w4389) -> (1/x=w4390:sgl)
                                n1622 = Bundle By Name("Y"=w4384, "dt"=w4390) -> (w4381:waveform(sgl))  [unwired: 1 in]
                                n1623 = call-poly <vilib>:"Analog to Digital.vi"("data format (offset binary)"=w4383, "compress digital (T)"=TRUE, "full-scale range (pk-pk)"=1.0, "resolution (16 bit)"=1, "analog waveform"=w4381) -> ("digital waveform"=w4380:digitalwaveform)  [unwired: 3 in, 3 out]
                                }
                                frame True {
                                w4396 = u16 0 items=["unsigned binary", "offset binary", "2's complement"] ("data format (offset binary)")
                                n1624 = To Double Precision Float(number=w4399) -> (double precision float=w4406:dbl)
                                n1625 = Initialize Array(sgl 0.0, w4399) -> (w4401:sgl[])
                                n1626 = Divide(x=w4405, y=w4406) -> (x/y=w4403:dbl)
                                n1627 = Round Toward +Infinity(x=w4403) -> (ceil(x): smallest int >= x=w4404:dbl)
                                n1628 = Replace Array Subset(array=w4401, new element=sgl 1.0, index=0) -> (w4398:sgl[])
                                n1629 = for {
                                N: w4404 -> [_]
                                tunnel: w4398 -> [w4410]
                                tunnel: [w4410] -> w4407 mode=concatenating
                                }
                                n1630 = Reciprocal(x=w4408) -> (1/x=w4409:sgl)
                                n1631 = Bundle By Name("Y"=w4407, "dt"=w4409) -> (w4394:waveform(sgl))  [unwired: 1 in]
                                n1632 = call-poly <vilib>:"Analog to Digital.vi"("data format (offset binary)"=w4396, "compress digital (T)"=TRUE, "full-scale range (pk-pk)"=1.0, "resolution (16 bit)"=1, "analog waveform"=w4394) -> ("digital waveform"=w4393:digitalwaveform)  [unwired: 3 in, 3 out]
                                }
                                }
                                n1633 = Build Array(w4367) -> (w4364:digitalwaveform[])
                                n1634 = Replace Array Subset(array=w4366, new element=w4370, index=w4365) -> (w4363:digitalwaveform[])
                                n1635 = call "waveformsDObuffer.vi"("DO wf in"=w4363, "command"="set") -> ()  [unwired: 1 out]
                                }
                                }
                                }
                                }
                                }
                                frame #10 {
                                n1636 = local read "Meastab"() -> (w4424:enum32{"X-Y Image", "Linescan", "Timetrace"})
                                n1637 = property on="refwf" class="Ring (strict)"() -> ("RingText.Text"=w4421:string)  [unwired: 2 in, 2 out]
                                n1638 = case shown="\"Timetrace\"" w4424 {
                                tunnel: [w4426 w4427] -> w4425
                                frame "X-Y Image", Default {
                                n1639 = local read "Sampling rate"() -> (w4426:dbl)
                                }
                                frame "Timetrace" {
                                n1640 = local read "srateAODOtt"() -> (w4427:dbl)
                                }
                                }
                                n1641 = call "waveformsAObuffer.vi"("command"="get") -> ("AO wf out"=w4414:waveform(dbl)[])  [unwired: 1 in]
                                n1642 = local read "wavdet"() -> (w4422:bool)
                                n1643 = call "waveformsDObuffer.vi"("command"="get") -> ("DO wf out"=w4418:digitalwaveform[])  [unwired: 1 in]
                                n1644 = call "correctwaveformsizetemp.vi"("new sampling frequency (Hz)"=w4425, "start"=TRUE, "reference waveforms to"=w4421, "Analog waveforms in"=w4414, "stop"=FALSE, "Digital waveforms in"=w4418) -> ("analog wf out"=w4420:waveform(dbl)[], "Digital wf out"=w4413:digitalwaveform[], "measpoints"=w4423:i32)
                                n1645 = call "waveformsDObuffer.vi"("DO wf in"=w4413, "command"="set") -> ()  [unwired: 1 out]
                                n1646 = call "waveformsAObuffer.vi"("AO wf in"=w4420, "command"="set") -> ()  [unwired: 1 out]
                                n1647 = case shown="True" w4422 {
                                tunnel: w4423 -> [_ w4430]
                                tunnel: w4413 -> [_ w4428]
                                frame False {
                                }
                                frame True {
                                n1648 = local write "# of frames"(w4430) -> ()
                                n1649 = call "GetNumCamFramesv2.vi"("Digital Waveform Graph"=w4428) -> ("Numeric"=w4429:i32)  [unwired: 10 in]
                                n1650 = local write "Total Camera Frames"(w4429) -> ()
                                }
                                }
                                }
                                }
                              }
                              frame #7 {
                                # "Disabled for conversion to 64 bit"
                                n1651 = disable-structure shown="Disabled" {
                                frame Disabled {
                                n1652 = local read "Measurement"() -> (w4432:T4)
                                n1653 = case shown="\"Lifetime (scan)\"" w4432 {
                                frame "X-Y-t movie", Default {
                                }
                                frame "Lifetime (scan)" {
                                # "total acquisition time"
                                n1654 = call "2pparameters.vi"("command"="get") -> ("params out"=w4440:T10)  [unwired: 1 in]
                                n1655 = Unbundle By Name(w4440) -> ("measpoints"=w4434:i32, "srateAODO"=w4455:sgl)
                                n1656 = Divide(x=w4434, y=w4455) -> (x/y=w4433:sgl)
                                n1657 = local read "min phot"() -> (w4450:u32)
                                n1658 = local read "expected c/s"() -> (w4451:dbl)
                                n1659 = Multiply(x=w4433, y=1000.0) -> (x*y=w4443:dbl)
                                n1660 = local read "Ch1 ZeroX"() -> (w4448:i32)
                                n1661 = local read "truncate"() -> (w4449:u32)
                                n1662 = To Long Integer(number=w4443) -> (32bit integer=w4452:i32)
                                n1663 = To Long Integer(number=w4451) -> (32bit integer=w4453:i32)
                                n1664 = local read "Number of Bins"() -> (w4444:u32)
                                n1665 = local read "Ch1 Level"() -> (w4446:i32)
                                n1666 = local read "Ch0 ZeroX"() -> (w4447:i32)
                                n1667 = local write "Acquisition time"(w4452) -> ()
                                n1668 = local read "Ch0 Level"() -> (w4445:i32)
                                n1669 = call "lifetimeparameters.vi"("command"="get") -> ("Params out"=w4438:T19)  [unwired: 1 in]
                                n1670 = Add(x=100, y=w4452) -> (x+y=w4442:i32)
                                n1671 = Bundle By Name(cluster=w4438, "acq time"=w4442, "acq rate"=w4453, "# bins"=w4444, "Ch0 Level"=w4445, "Ch1 Level"=w4446, "Ch0 ZeroX"=w4447, "Ch1 ZeroX"=w4448, "min photons"=w4450, "truncate"=w4449) -> (w4437:T19)
                                n1672 = local write "Acquisition rate"(w4453) -> ()
                                n1673 = call "lifetimeparameters.vi"("Params in"=w4437, "command"="set") -> ()  [unwired: 1 out]
                                }
                                }
                                }
                                frame Enabled {
                                }
                                }
                                n1674 = local write "64bit disabled"(TRUE ("64bit disabled")) -> ()
                              }
                              frame #8 {
                                n1675 = call "2pparameters.vi"("command"="get") -> ("params out"=w4466:T10)  [unwired: 1 in]
                                n1676 = Unbundle By Name(w4466) -> ("refreshbuffer"=w4464:i32, "srate"=w4465:sgl)
                                n1677 = local read "wavdet"() -> (w4456:bool)
                                n1678 = To Double Precision Float(number=w4465) -> (double precision float=w4468:dbl)
                                n1679 = To Double Precision Float(number=w4464) -> (double precision float=w4459:dbl)
                                n1680 = case shown="False" w4456 {
                                tunnel: [w4473 w4474] -> w4458
                                frame False {
                                w4473 = 10123 items=["Finite Samples"=10178, "Continuous Samples"=10123, "Hardware Timed Single Point"=12522] ("sample mode")
                                }
                                frame True {
                                w4474 = 10123 items=["Finite Samples"=10178, "Continuous Samples"=10123, "Hardware Timed Single Point"=12522] ("sample mode")
                                }
                                }
                                n1681 = Divide(x=w4459, y=w4468) -> (x/y=w4472:dbl)
                                n1682 = Multiply(x=w4472, y=2.0) -> (x*y=w4469:dbl)
                                n1683 = Max & Min(x=w4469, y=10.0) -> (max(x,y)=w4460:dbl)  [unwired: 1 out]
                                n1684 = call "2pparameters.vi"("command"="get") -> ("params out"=w4463:T10)  [unwired: 1 in]
                                n1685 = Bundle By Name(cluster=w4463, "timeout"=w4460, "sample mode"=w4458) -> (w4461:T10)
                                n1686 = call "2pparameters.vi"("Params in"=w4461, "command"="set") -> ()  [unwired: 1 out]
                              }
                            }
                          }
                          frame #1 {
                            # "Disabled for conversion to 64 bit"
                            n1687 = call "prepAO_img.vi"() -> ("Terminal Name with Device Prefix"=w4476:tag)
                            n1688 = call "prepDO_img.vi"() -> ()  [unwired: 2 in]
                            n1689 = call "prepAI_img.vi"("triggersource"=w4476) -> ()  [unwired: 2 in]
                            n1690 = call "prepCI_img.vi"("ArmStart.DigEdge.Src"=w4476) -> ()  [unwired: 1 in]
                            n1691 = disable-structure shown="Disabled" {
                              frame Disabled {
                                n1692 = local read "Measurement"() -> (w4477:T4)
                                n1693 = case shown="\"Lifetime (contour)\"" w4477 {
                                frame "X-Y-t movie", Default {
                                }
                                frame "Lifetime (contour)" {
                                n1694 = stacked-sequence {
                                frame #0 {
                                n1695 = call "PH-temp.vi"("String"="clear" ("command")) -> ()  [unwired: 2 in, 2 out]
                                n1696 = call "PH-temp-raw.vi"("command"="empty") -> ()  [unwired: 1 in, 1 out]
                                }
                                frame #1 {
